vi "TEMP.vi"() -> ()   [LabVIEW 2025]
panel:
  out "Boolean":bool
  out "output":string
  out "iteration":dbl
  in  "stop":bool
  out "Thermometer":dbl(slide) scale=0.0..100.0
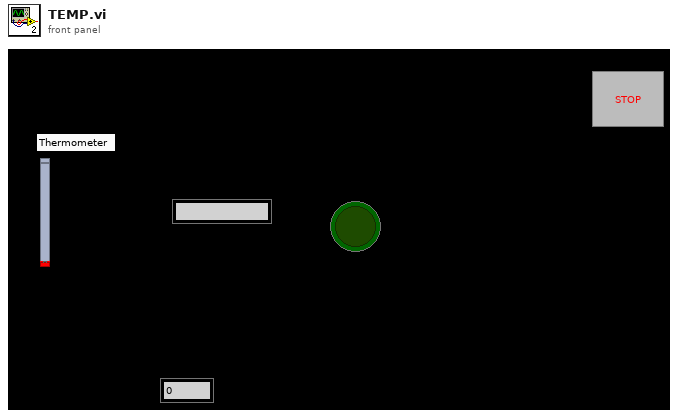
[diagram p1: front panel]
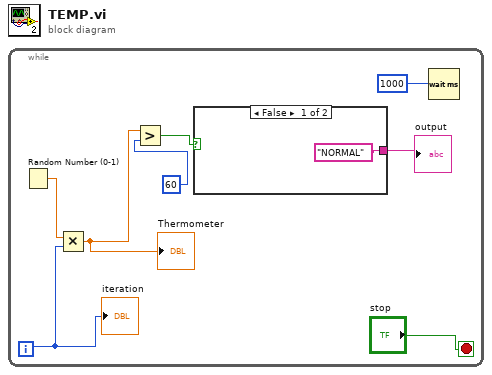
[diagram p0: block diagram]
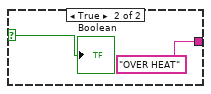
[diagram p2: hidden frame]
diagram:
  n1 = while {
    i -> [w6]
    stop <- "stop" stop-if-true
    n2 = Random Number (0-1)() -> (number: 0 to 1=w7:dbl)
    n3 = Multiply(x=w7, y=w6) -> (x*y=w4:dbl)
    "Thermometer" <- w4
    n4 = Greater?(x=w4, y=60) -> (0:w1:bool)
    n5 = case shown="False" w1 {
      selector: w1 -> [_ w10]
      tunnel: ["NORMAL" "OVER HEAT"] -> w3
      frame False {
      }
      frame True {
        "Boolean" <- w10
      }
    }
    "output" <- w3
    n6 = Wait (ms)(milliseconds to wait=1000) -> ()  [unwired: 1 out]
    "iteration" <- w6
  }
